vi "server.vi"() -> ()   [LabVIEW 2015]
uses:
  Global/SeverGlobal.vi
panel:
  in  "stop":bool
  out "Connect":i32
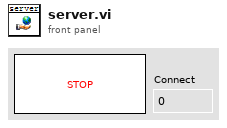
[diagram p1: front panel]
types:
  T1 = typedef "队列.ctl" = cluster{"COM1":refnum<queue>, "COM2":refnum<queue>, "COM3":refnum<queue>, "COM4":refnum<queue>, "OUT1":refnum<queue>, "OUT2":refnum<queue>, "OUT3":refnum<queue>, "OUT4":refnum<queue>, "OUT5":refnum<queue>, "OUT6":refnum<queue>, "OUT7":refnum<queue>, "OUT8":refnum<queue>}
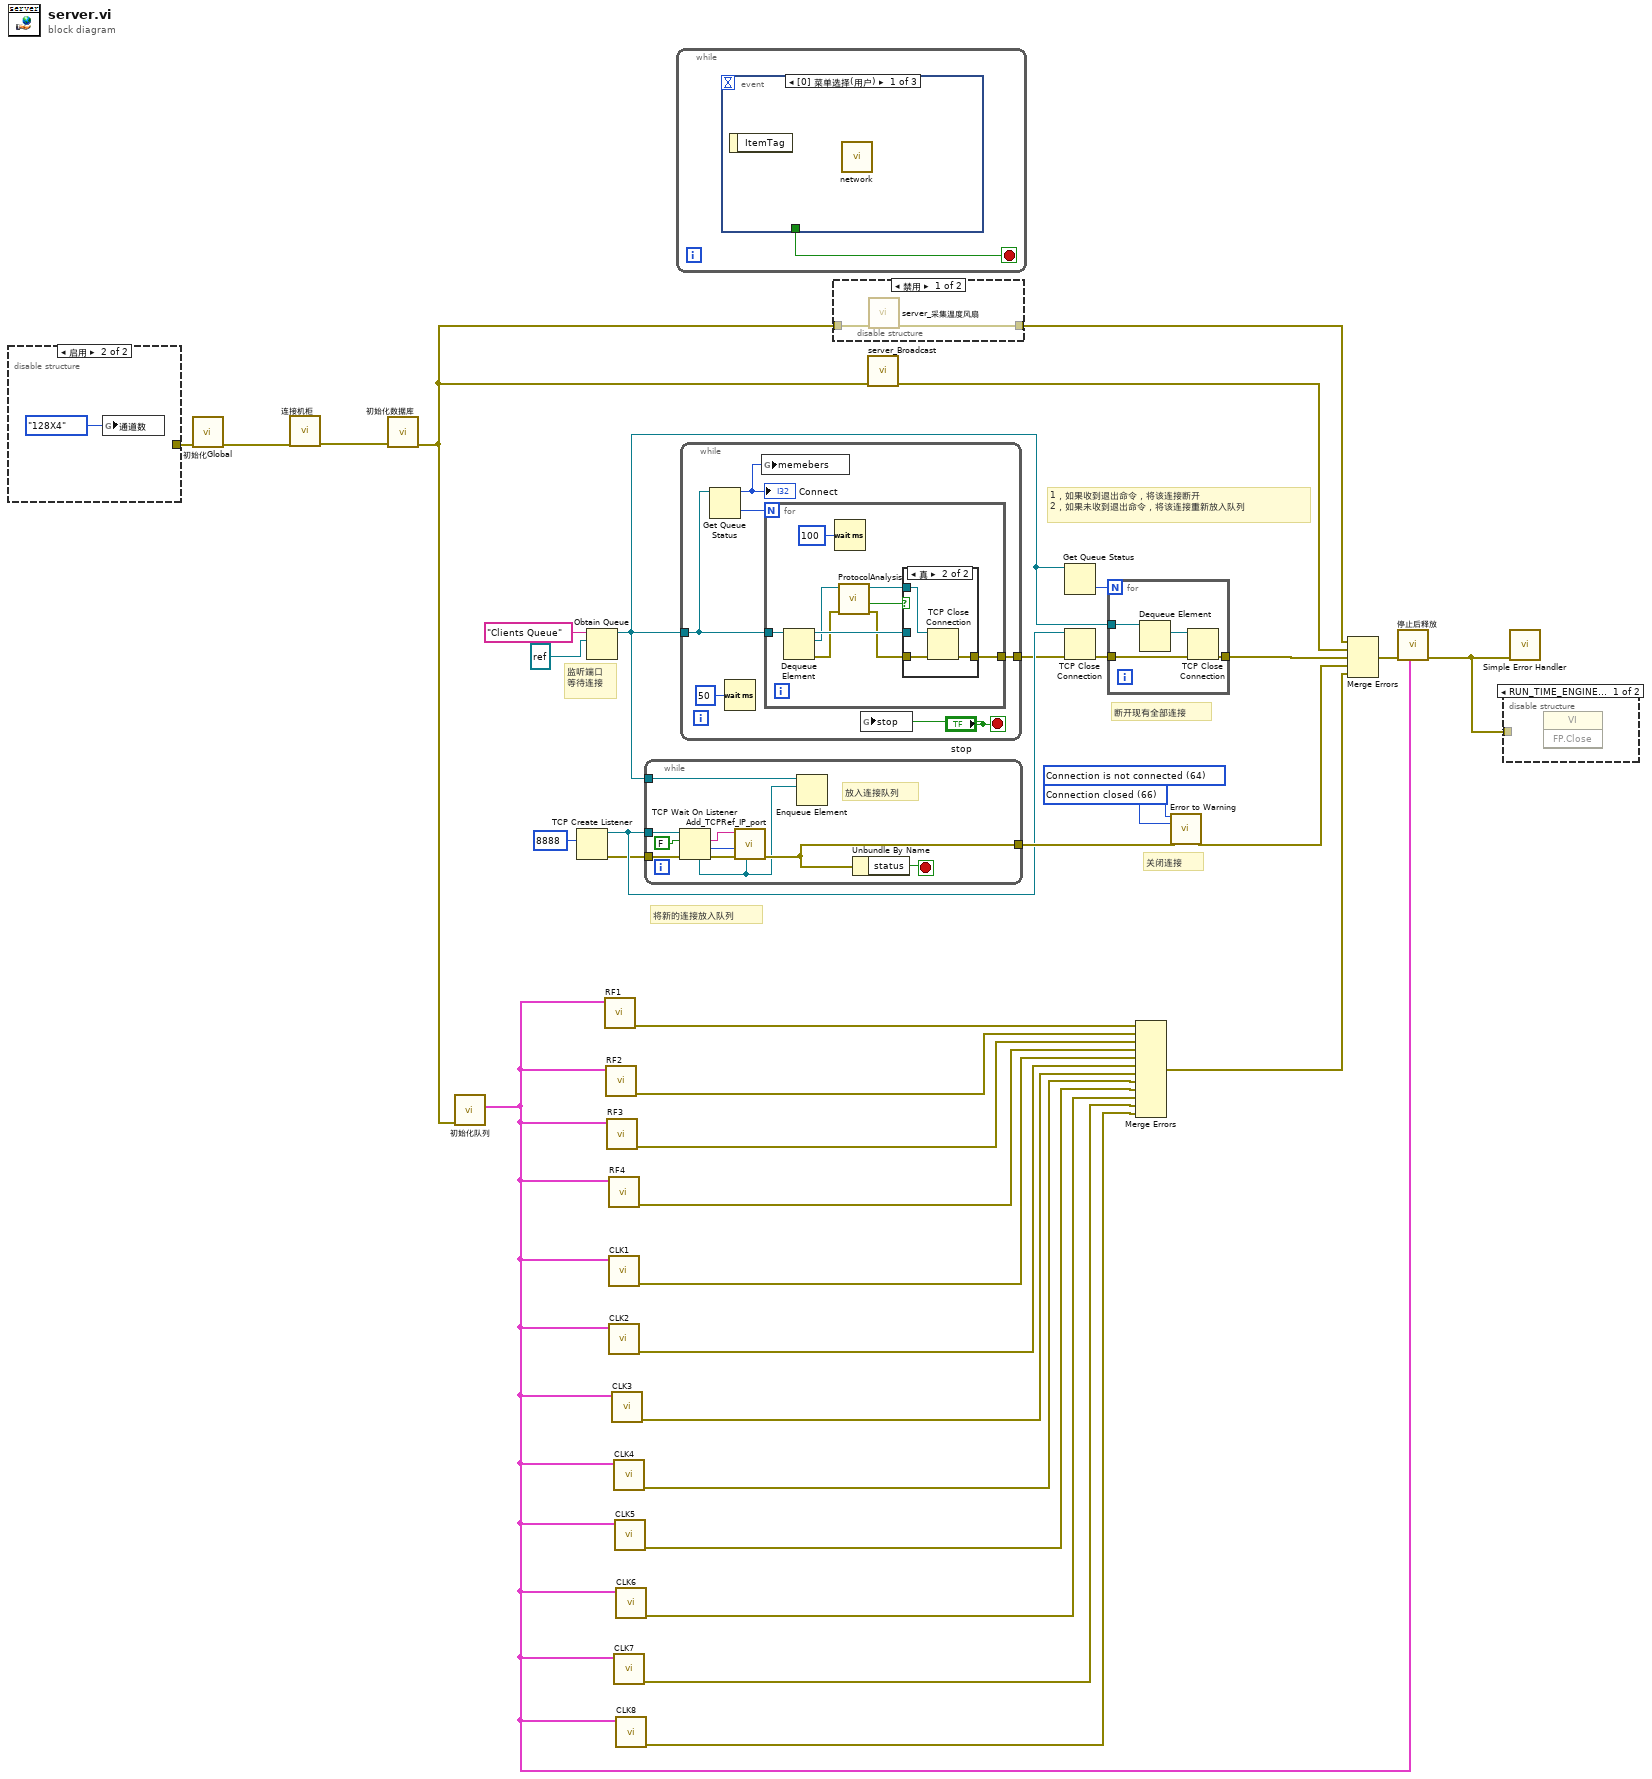
[diagram p0: block diagram]
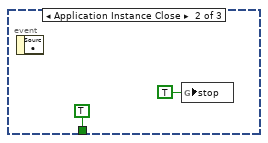
[diagram p2: hidden frame]
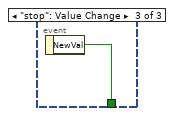
[diagram p3: hidden frame]
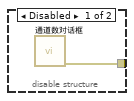
[diagram p4: hidden frame]
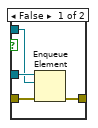
[diagram p7: hidden frame]
diagram:
  w26 = 66 items=["No Error", "Argument Error", "Memory Full", "Out of Zone", "End of File", "File Already Open", "Generic File IO Error", "File Not Found", "File Permission Error", "Disk Full", "Duplicate Path", "Too Many Files Open", "Not Enabled", "Resource File Not Found", "Cannot Add Resource", "Resource Not Found", "Image Not Found", "Image Memory Error", "Pen Does Not Exist", "Config Bad Type", "Config Token Not Found", "Config Parse Error", "Config Memory Error", "Bad External Code Format", "Bad External Code Offset", "External Code Not Present", "Null Window", "Destroy Window Mixup", "Null Menu", "Print Aborted", "Bad Print Record", "Print Driver Error", "Windows Error During Print", "Memory Error During Print", "Print Dialog Error", "Generic Print Error", "Invalid Device Refnum", "Device Not Found", "Device Parameter Error", "Device Unit Error", "Can't Open Device", "Device Call Aborted", "Generic Error", "Cancelled By User", "Object ID Too Low", "Object ID Too High", "Object Not In Heap", "Unknown Heap", "Bad DefProc ID", "DefProc Not In Table", "Message Out Of Range", "Null Method", "Unknown Message", "Manager Call Not Supported", "Bad address", "Connection In progress", "Connection timed out", "Connection is already in progress", "Network attribute not supported", "Network error", "Address in use", "System out of memory", "Connection aborted", "Connection refused", "Connection is not connected", "Connection is already connected", "Connection closed", "Initialize error (interapplication manager)", "Bad occurrence", "Wait on unbound occurrence handler", "Occurrence queue overflow", "Bad path", "Semaphore not signaled", "Unrecognized type (interapplication manager)"] ("2nd Error to Convert")
  w25 = 64 items=["No Error", "Argument Error", "Memory Full", "Out of Zone", "End of File", "File Already Open", "Generic File IO Error", "File Not Found", "File Permission Error", "Disk Full", "Duplicate Path", "Too Many Files Open", "Not Enabled", "Resource File Not Found", "Cannot Add Resource", "Resource Not Found", "Image Not Found", "Image Memory Error", "Pen Does Not Exist", "Config Bad Type", "Config Token Not Found", "Config Parse Error", "Config Memory Error", "Bad External Code Format", "Bad External Code Offset", "External Code Not Present", "Null Window", "Destroy Window Mixup", "Null Menu", "Print Aborted", "Bad Print Record", "Print Driver Error", "Windows Error During Print", "Memory Error During Print", "Print Dialog Error", "Generic Print Error", "Invalid Device Refnum", "Device Not Found", "Device Parameter Error", "Device Unit Error", "Can't Open Device", "Device Call Aborted", "Generic Error", "Cancelled By User", "Object ID Too Low", "Object ID Too High", "Object Not In Heap", "Unknown Heap", "Bad DefProc ID", "DefProc Not In Table", "Message Out Of Range", "Null Method", "Unknown Message", "Manager Call Not Supported", "Bad address", "Connection In progress", "Connection timed out", "Connection is already in progress", "Network attribute not supported", "Network error", "Address in use", "System out of memory", "Connection aborted", "Connection refused", "Connection is not connected", "Connection is already connected", "Connection closed", "Initialize error (interapplication manager)", "Bad occurrence", "Wait on unbound occurrence handler", "Occurrence queue overflow", "Bad path", "Semaphore not signaled", "Unrecognized type (interapplication manager)"] ("1st Error to Convert")
  # "断开现有全部连接"
  # "1，如果收到退出命令，将该连接断开\n2，如果未收到退出命令，将该连接重新放入队列"
  # "将新的连接放入队列"
  # "关闭连接"
  # "监听端口\n等待连接"
  n1 = disable-structure shown="启用" {
    disable-tunnel: [w37 _] -> w2
    frame Disabled {
      n2 = call "通道数对话框.vi"() -> ("error out"=w37:errorcluster)  [unwired: 11 in]
    }
    frame Enabled {
      n3 = global write "SeverGlobal.vi" "通道数"(enum16{"64X4", "128X4"}."128X4" ("Channel count")) -> ()
    }
  }
  n4 = call "初始化Global.vi"("error in (no error)"=w2) -> ("error out"=w22:errorcluster)  [unwired: 10 in]
  n5 = call "连接机柜.vi"("error in (no error)"=w22) -> ("error out"=w23:errorcluster)  [unwired: 10 in]
  n6 = call "初始化数据库.vi"("error in (no error)"=w23) -> ("error out"=w1:errorcluster)  [unwired: 10 in]
  n7 = call "初始化队列.vi"("error in (no error)"=w1) -> ("Queue Out"=w5:T1)  [unwired: 9 in, 1 out]
  n8 = TCP Create Listener(10:u32 8888 ("端口")) -> (0:w27:errorcluster, 3:w28:refnum<k5>)  [unwired: 4 in, 1 out]
  n9 = Obtain Queue(name (unnamed)="Clients Queue", element data type=refnum<k5> refnum ("listener ID out")) -> (queue out=w36:refnum<queue>)  [unwired: 3 in, 2 out]
  n10 = call "RF1.vi"("Queue Out"=w5) -> ("error out"=w17:errorcluster)  [unwired: 10 in]
  n11 = call "RF2.vi"("Queue Out"=w5) -> ("error out"=w15:errorcluster)  [unwired: 10 in]
  n12 = call "RF3.vi"("Queue Out"=w5) -> ("error out"=w14:errorcluster)  [unwired: 10 in]
  n13 = call "RF4.vi"("Queue Out"=w5) -> ("error out"=w13:errorcluster)  [unwired: 10 in]
  n14 = call "CLK1.vi"("Queue Out"=w5) -> ("error out"=w12:errorcluster)  [unwired: 10 in]
  n15 = call "CLK2.vi"("Queue Out"=w5) -> ("error out"=w11:errorcluster)  [unwired: 10 in]
  n16 = call "CLK3.vi"("Queue Out"=w5) -> ("error out"=w10:errorcluster)  [unwired: 10 in]
  n17 = call "CLK4.vi"("Queue Out"=w5) -> ("error out"=w9:errorcluster)  [unwired: 10 in]
  n18 = call "CLK7.vi"("Queue Out"=w5) -> ("error out"=w6:errorcluster)  [unwired: 10 in]
  n19 = call "CLK5.vi"("Queue Out"=w5) -> ("error out"=w8:errorcluster)  [unwired: 10 in]
  n20 = call "CLK6.vi"("Queue Out"=w5) -> ("error out"=w7:errorcluster)  [unwired: 10 in]
  n21 = call "CLK8.vi"("Queue Out"=w5) -> ("error out"=w4:errorcluster)  [unwired: 10 in]
  n22 = while {
    tunnel: w28 -> [w48]
    tunnel: w27 -> [w47]
    tunnel: [w43] -> w30
    tunnel: w36 -> [w45]
    stop <- w46 stop-if-true
    # "放入连接队列"
    n23 = TCP Wait On Listener(8:w47, 10:FALSE ("resolve remote address (T)"), 11:w48) -> (0:w44:errorcluster, 1:w40:u16, 2:w41:string, 4:w42:refnum<k5>)  [unwired: 1 in, 1 out]
    n24 = call "Add_TCPRef_IP_port.vi"("TCP Ref"=w42, "error in"=w44, "port"=w40, "IP"=w41) -> ("error out"=w43:errorcluster)  [unwired: 7 in]
    n25 = Enqueue Element(queue=w45, element=w42) -> ()  [unwired: 2 in, 3 out]
    n26 = Unbundle By Name(w43) -> ("status"=w46:bool)
  }
  n27 = while {
    stop <- w49 stop-if-true
    n28 = event shown="[0] 菜单选择(用户)" {
      selector: _ -> [_ _ _]
      dyn-events: _ -> [_ _ _]
      timeout: _ -> [_ _ _]
      tunnel: [_ TRUE ("NewVal") w52] -> w49
      event Menu Selection (User) {
        n29 = event-data() -> ()  [unwired: 1 in, 1 out]
        n30 = call "network.vi"() -> ()  [unwired: 20 in]
      }
      event Application Instance Close {
        n31 = event-data() -> ()  [unwired: 1 in, 1 out]
        n32 = global write "SeverGlobal.vi" "stop"(TRUE ("stop")) -> ()
      }
      event "stop": Value Change {
        n33 = event-data() -> ("NewVal"=w52:bool)  [unwired: 1 in]
      }
    }
  }
  n34 = while {
    tunnel: [w57] -> w24
    tunnel: w36 -> [w56]
    stop <- "stop" stop-if-true
    n35 = Get Queue Status(queue=w56) -> (# elements in queue=w54:i32)  [unwired: 2 in, 7 out]
    "Connect" <- w54
    n36 = Wait (ms)(milliseconds to wait=u32 50 ("等待时间（毫秒）")) -> ()  [unwired: 1 out]
    n37 = global write "SeverGlobal.vi" "memebers"(w54) -> ()
    n38 = for {
      N: w54 -> [_]
      tunnel: [w64] -> w57
      tunnel: w56 -> [w66]
      n39 = Dequeue Element(queue=w66) -> (queue out=w65:refnum<queue>, element=w63:refnum<k5>, error out=w62:errorcluster)  [unwired: 2 in, 1 out]
      n40 = Wait (ms)(milliseconds to wait=u32 100 ("等待时间（毫秒）")) -> ()  [unwired: 1 out]
      n41 = call "ProtocolAnalysis.vi"("error in"=w62, "IP"=w63) -> ("error out"=w60:errorcluster, "Disconnected"=w59:bool, "IP 2"=w61:refnum<k5>)  [unwired: 7 in]
      n42 = case shown="真" w59 {
        tunnel: w65 -> [w70 _]
        tunnel: [w69 w71] -> w64
        tunnel: w61 -> [w68 w73]
        tunnel: w60 -> [w67 w72]
        frame False {
          n43 = Enqueue Element(queue=w70, element=w68, error in (no error)=w67) -> (error out=w69:errorcluster)  [unwired: 1 in, 2 out]
        }
        frame True {
          n44 = TCP Close Connection(connection ID=w73, error in (no error)=w72) -> (error out=w71:errorcluster)  [unwired: 1 in, 1 out]
        }
      }
    }
    n45 = global write "SeverGlobal.vi" "stop"("stop") -> ()
  }
  n46 = disable-structure shown="禁用" {
    disable-tunnel: [w75 w76] -> w3
    disable-tunnel: w1 -> [w74 w76]
    frame Disabled {
      n47 = call "server_采集温度风扇.vi"("error in (no error)"=w74) -> ("error out"=w75:errorcluster)  [unwired: 10 in]
    }
    frame Enabled {
    }
  }
  n48 = call "server_Broadcast.vi"("错误输入（无错误）"=w1) -> ("error out"=w21:errorcluster)  [unwired: 10 in]
  n49 = Get Queue Status(queue=w36) -> (# elements in queue=w34:i32)  [unwired: 2 in, 7 out]
  n50 = TCP Close Connection(connection ID=w28, error in (no error)=w24) -> (error out=w29:errorcluster)  [unwired: 1 in, 1 out]
  n51 = for {
    N: w34 -> [_]
    tunnel: w29 -> [w80]
    tunnel: [w79] -> w20
    tunnel: w36 -> [w78]
    n52 = Dequeue Element(queue=w78) -> (element=w77:refnum<k5>)  [unwired: 2 in, 3 out]
    n53 = TCP Close Connection(connection ID=w77, error in (no error)=w80) -> (error out=w79:errorcluster)  [unwired: 1 in, 1 out]
  }
  n54 = Merge Errors(w17, w15, w14, w13, w12, w11, w10, w9, w8, w7, w6, w4) -> (w16:errorcluster)
  n55 = call <vilib>:"Error to Warning.vi"("1st Error to Convert"=w25, "2nd Error to Convert"=w26, "error in"=w30) -> ("warning out"=w31:errorcluster)  [unwired: 12 in]
  n56 = Merge Errors(w3, w21, w20, w31, w16) -> (w19:errorcluster)
  n57 = call "停止后释放.vi"("Queue In"=w5, "error in (no error)"=w19) -> ("error out"=w18:errorcluster)  [unwired: 9 in]
  n58 = disable-structure shown="RUN_TIME_ENGINE==True" {
    disable-tunnel: w18 -> [_ _]
    frame condition #0 {
      n59 = invoke class="VI" method="FP.Close"() -> ()  [unwired: 3 in, 3 out]
    }
    frame condition #1 (active) {
    }
  }
  n60 = call <vilib>:"Simple Error Handler.vi"("error in (no error)"=w18) -> ()  [unwired: 4 in, 5 out]
